vi "3d_display4.vi"() -> ()   [LabVIEW 2009]
doc: "This example demonstrates some fundamental concepts for the 3D picture control. Concepts covered include:\n\n-Object creation\n-Texturing\n-Object movement\n-Object hierarchy"
uses:
  labWOOOO/wiimotestate.ctl
  labWOOOO/wiimoteState(IR).ctl
  <vilib>/Utility/miscctls.llb/LVRectTypeDef.ctl
  <vilib>/Utility/miscctls.llb/LV3DPointTypeDef.ctl
  C:/Documents and Settings/pbooth/My Documents/labWOOOO/WiimoteLib.dll
  <vilib>/picture/3D Picture Control/NI_3D Picture Control.lvlib
  <vilib>/Analysis/NI_AALBase.lvlib
panel:
  out "Boolean":bool
  out "element x":sgl
  out "element y":sgl
  out "Cluster":cluster{"Wiimote State":T1, "IRState":T2} {"IRState"."Mode" items=["Off"=0, "Basic"=1, "Extended"=3, "Full"=5]}
  out "xadd":dbl
  out "zadd":dbl
  out "raw pitot":dbl
  in  "Calibrate pitot":bool
  in  "voltage offset":dbl=2.5
  in  "velocity scale":dbl=100.0
  in  "Set Start Time (s)":dbl
  in  "X":dbl
  in  "Z":dbl
  in  "Calibrate Z":bool
  in  "Calibrate Y":bool
  in  "Calibrate X":bool
  out "angle 2":dbl
  out "angle 1":dbl
  out "X mean acceleration":dbl format="%0.4f"
  out "Y mean acceleration":dbl format="%0.4f"
  out "X mean volts":dbl format="%0.4f"
  out "Y mean volts":dbl format="%0.4f"
  out "Z mean acceleration":dbl format="%0.4f"
  out "Z mean volts":dbl format="%0.4f"
  in  "z gain":dbl=5.0
  in  "z offset":dbl=1.25
  in  "y gain":dbl=5.0
  in  "y offset":dbl=1.25
  in  "x gain":dbl=5.0
  in  "x offset":dbl=1.25
  in  "Render Dest":enum16{"Scene Window", "Scene Display"}(ring)
  in  "Camera Controller":enum16{"None", "Spherical", "Flying"}(ring)=enum."Spherical"
  out "Scene Display":refnum<vi>(3d-picture)
  in  "stop":bool
  # "Accelerometers"
  # "Buttons"
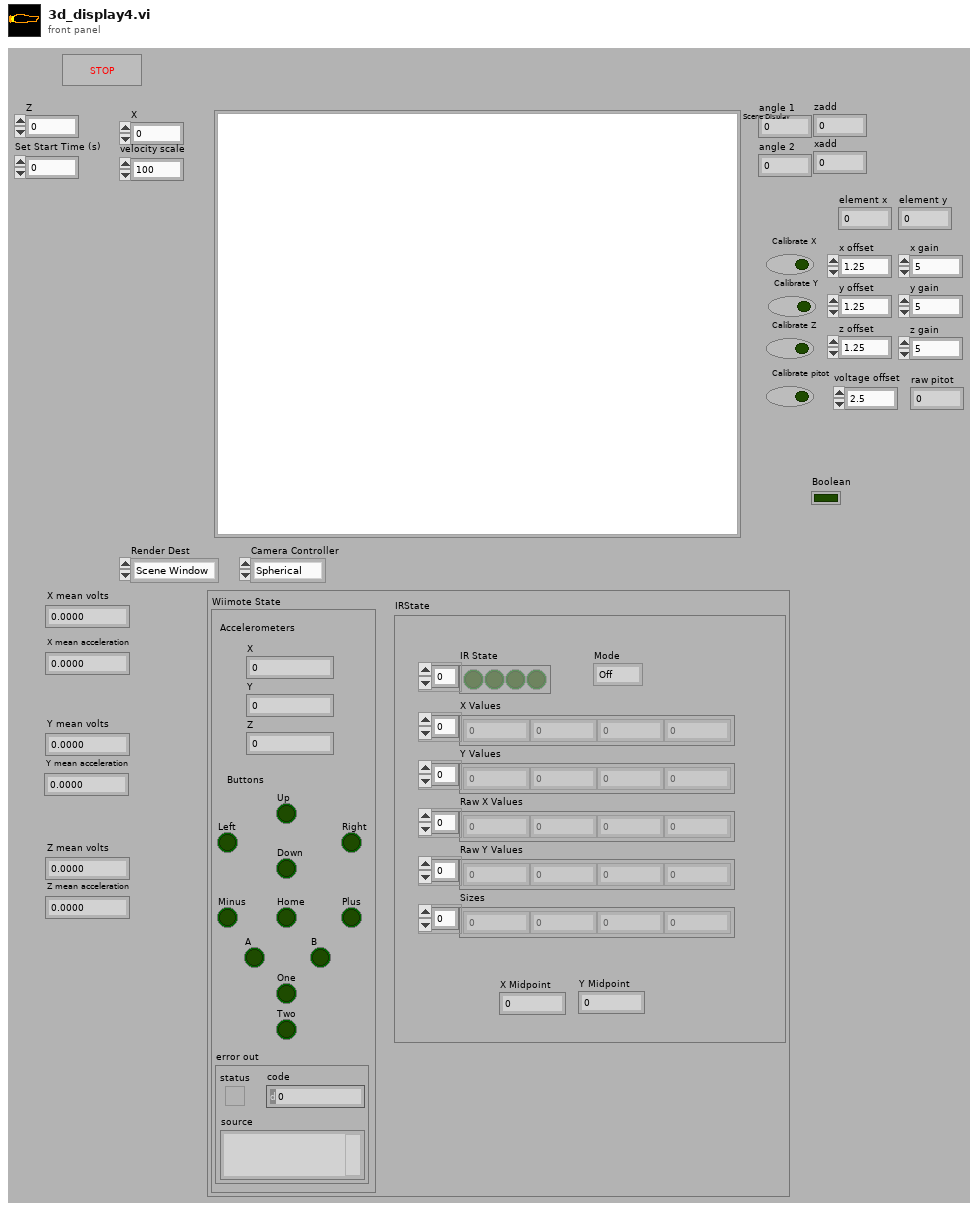
[diagram p1: front panel]
types:
  T1 = typedef "wiimotestate.ctl" = cluster{"X":sgl, "Y":sgl, "Z":sgl, "A":bool, "B":bool, "Down":bool, "Home":bool, "Left":bool, "Minus":bool, "One":bool, "Plus":bool, "Right":bool, "Two":bool, "Up":bool, "error out":errorcluster}
  T2 = typedef "wiimoteState(IR).ctl" = cluster{"Mode":u8, "IR State":bool[], "X Values":sgl[], "Y Values":sgl[], "Raw X Values":i32[], "Raw Y Values":i32[], "Sizes":i32[], "X Midpoint":sgl, "Y Midpoint":sgl}
  T3 = enum16{"As a Decal", "With Modulation", "With Blending", "As a replacement"}
  T4 = typedef "LVRectTypeDef.ctl" = cluster{"Left":i16, "Top":i16, "Right":i16, "Bottom":i16}
  T5 = enum16{"Open", "Minimized", "Maximized", "Hidden"}
  T6 = typedef "imagedata.ctl" = cluster{"image type":i32, "image depth":i32, "image":u8[], "mask":u8[], "colors":u32[], "Rectangle":cluster{"left":i16, "top":i16, "right":i16, "bottom":i16}}
  T7 = typedef "LV3DPointTypeDef.ctl" = cluster{"X":sgl, "Y":sgl, "Z":sgl}
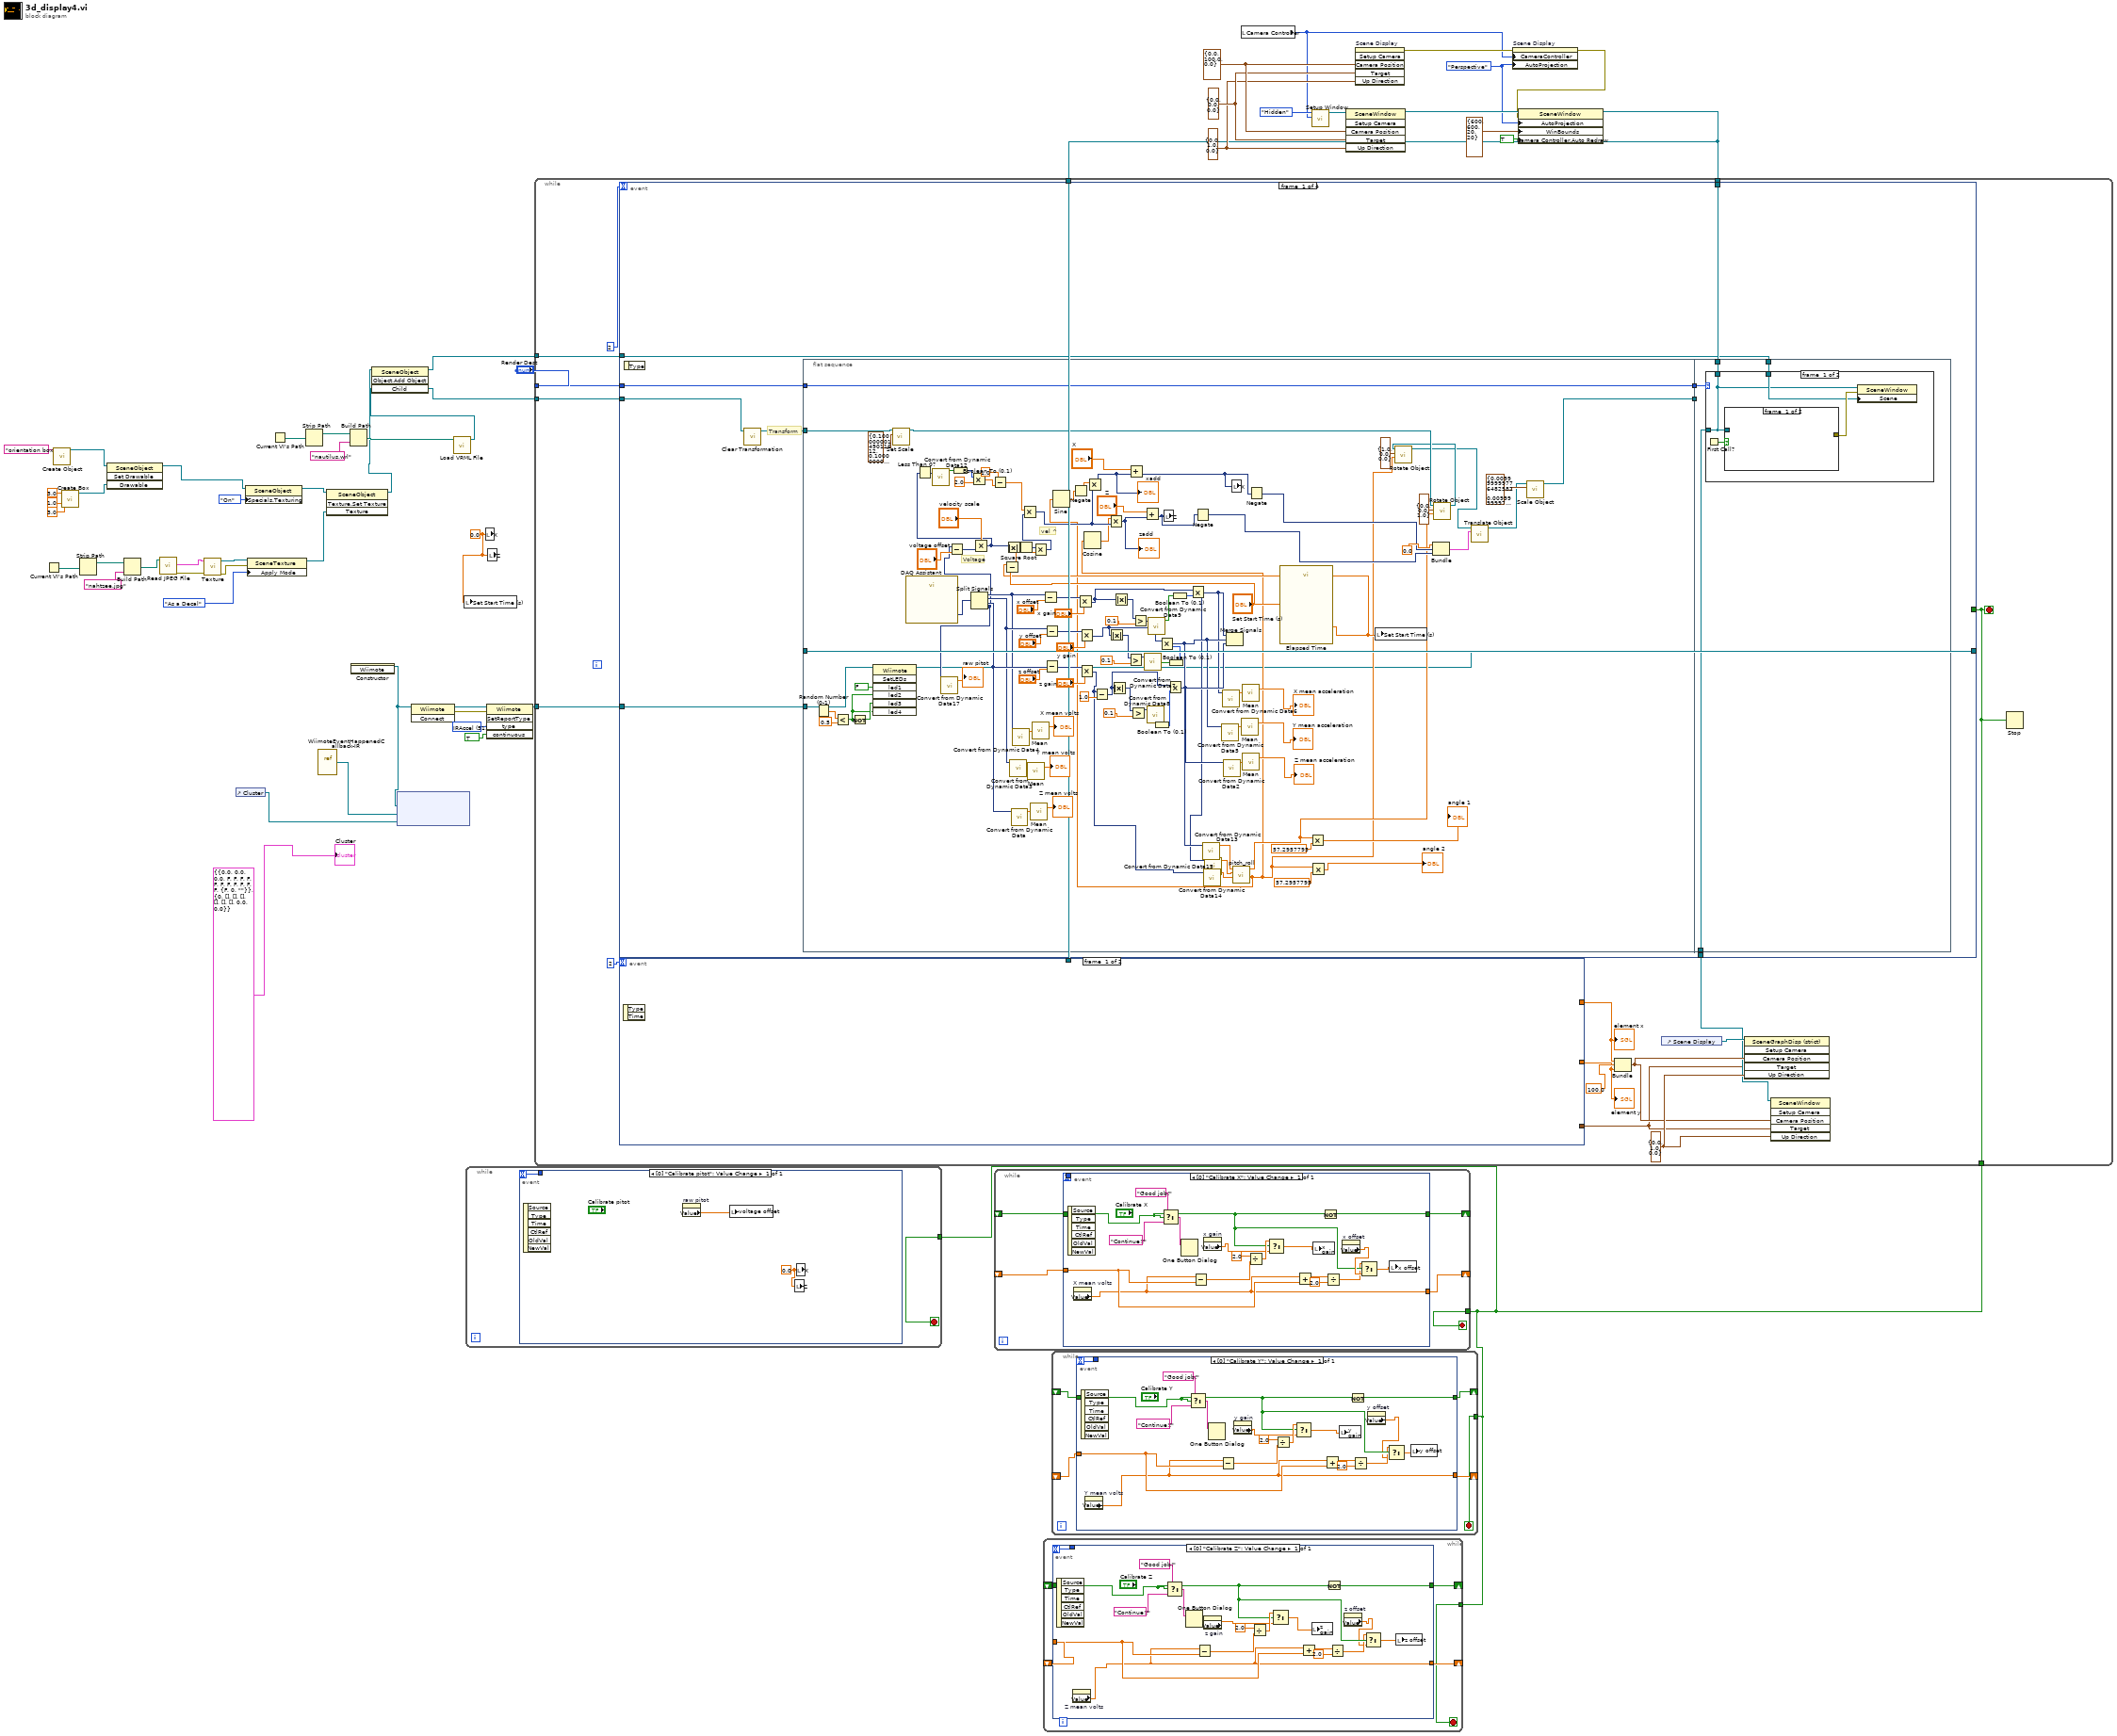
[diagram p0: block diagram]
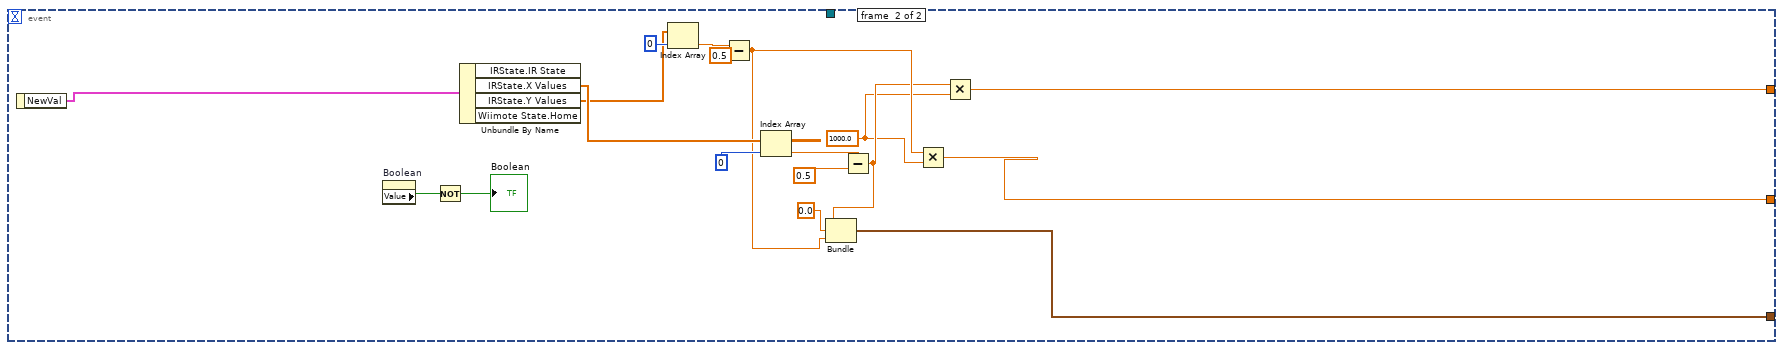
[diagram p2: hidden frame]
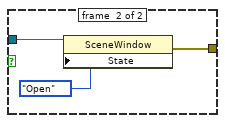
[diagram p3: hidden frame]
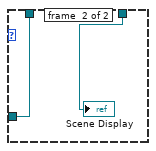
[diagram p4: hidden frame]
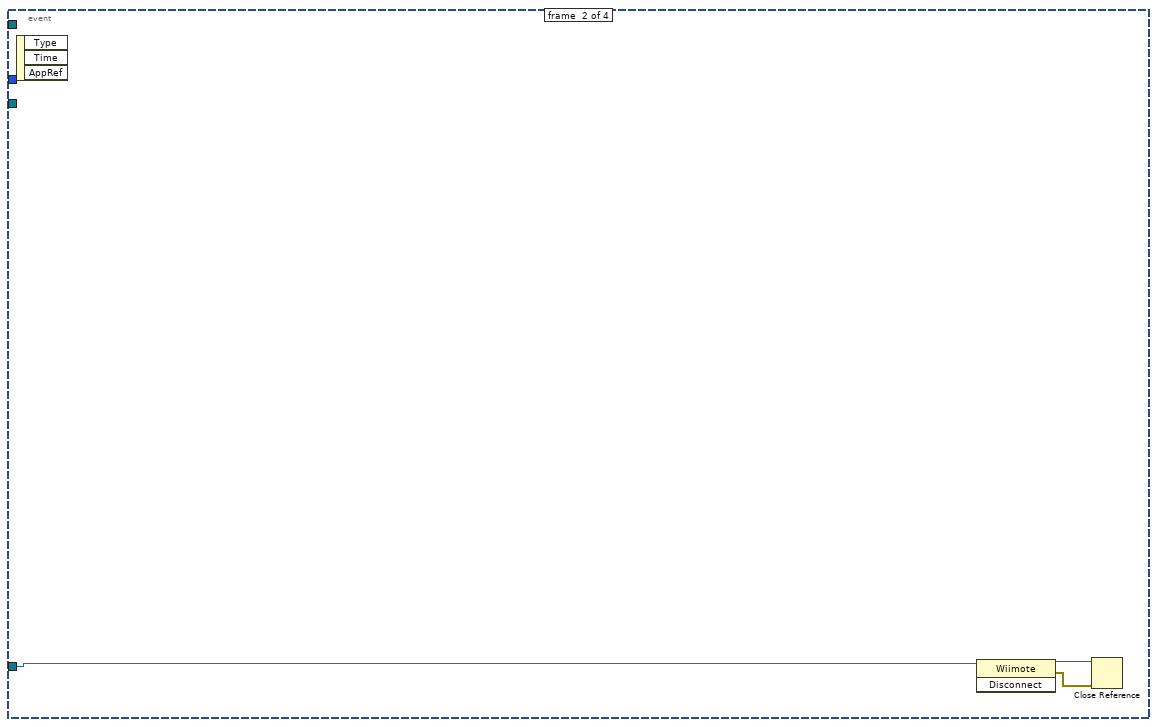
[diagram p5: hidden frame]
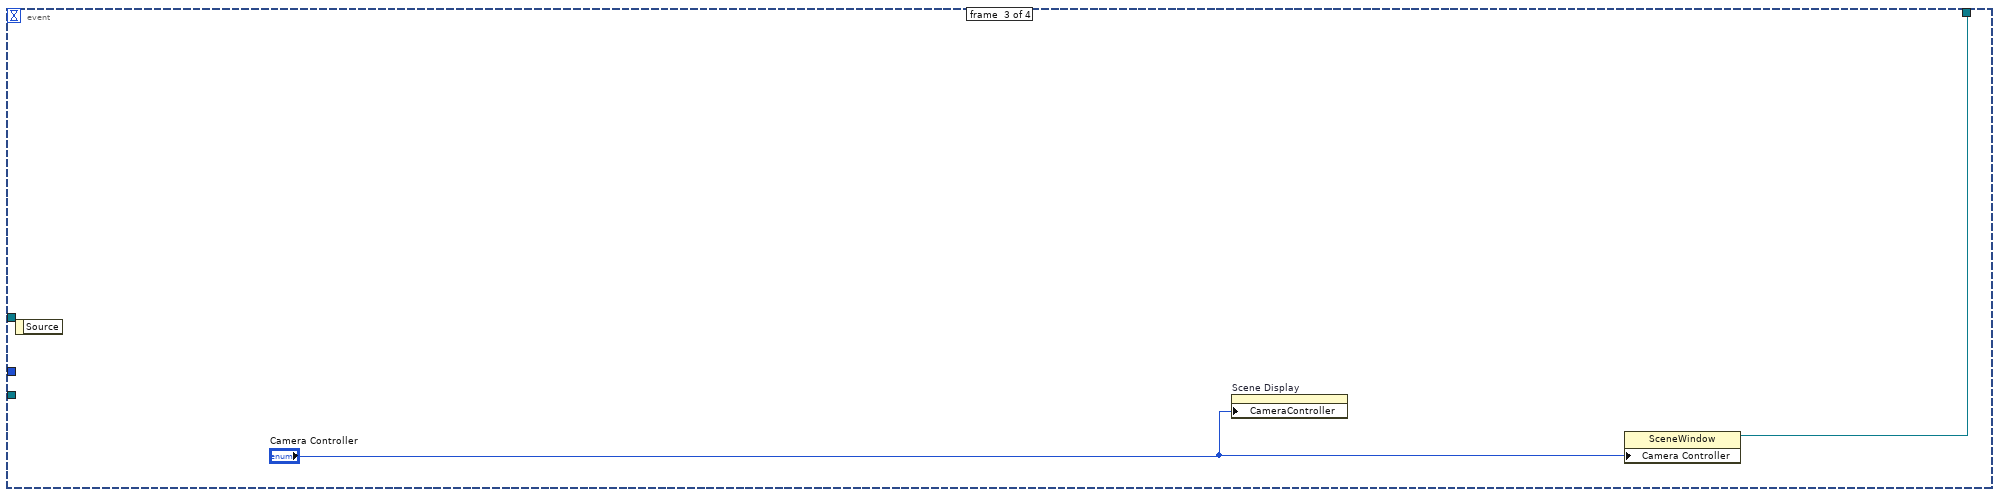
[diagram p6: hidden frame]
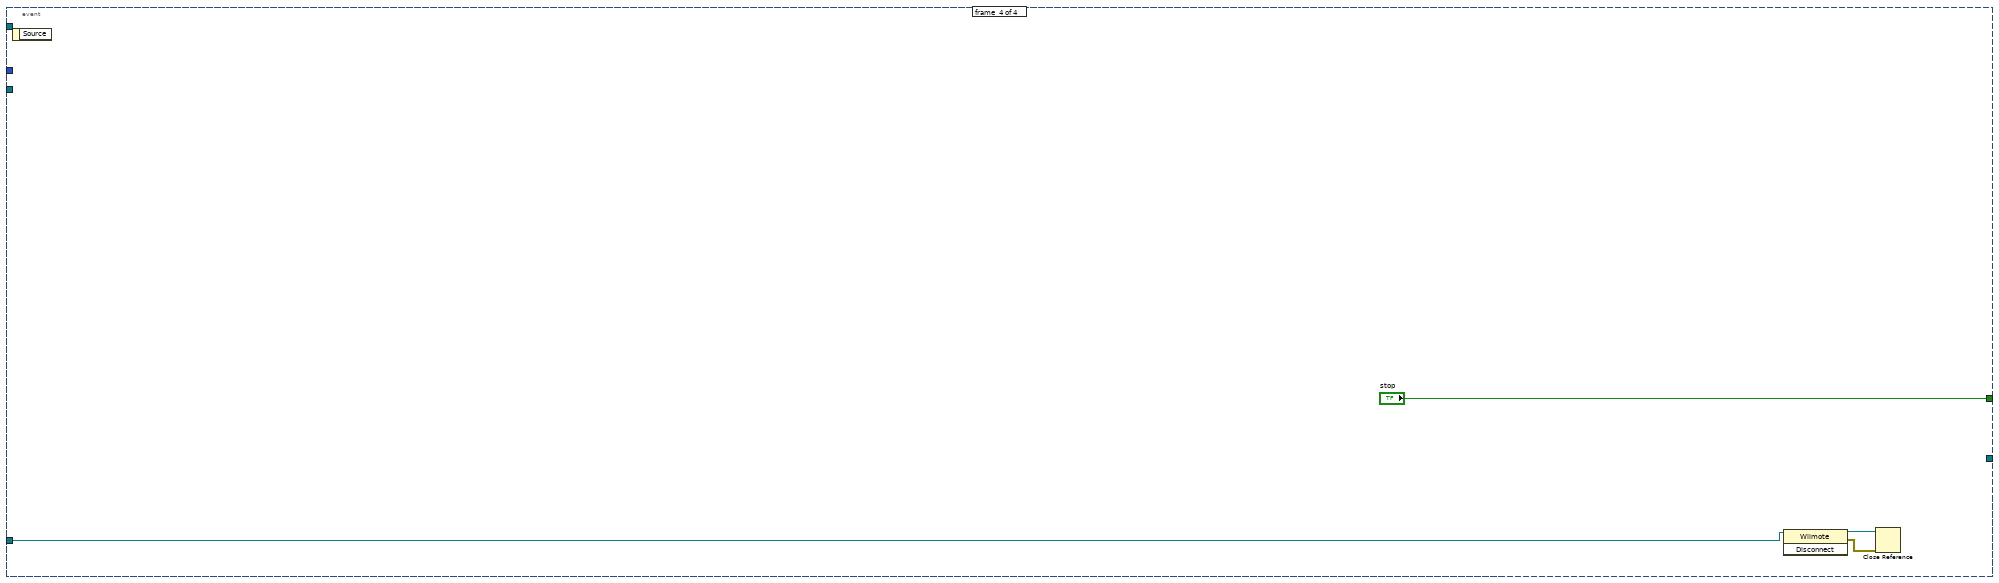
[diagram p7: hidden frame]
diagram:
  w28 = u8 51 items=["Status"=32, "ReadData"=33, "Buttons"=48, "ButtonsAccel"=49, "IRAccel"=51, "ButtonsExtension"=52, "ExtensionAccel"=53, "IRExtensionAccel"=55] ("type")
  w35 = 0.0 ("X")
  w45 = enum16{"None", "Perspective", "Orthographic"}."Perspective" ("Auto Projection Mode")
  w48 = cluster{"X":sgl, "Y":sgl, "Z":sgl} {"X"=0.0, "Y"=1.0, "Z"=0.0} ("Up Direction")
  w49 = cluster{"X":sgl, "Y":sgl, "Z":sgl} {"X"=0.0, "Y"=0.0, "Z"=0.0} ("Target")
  w50 = cluster{"X":sgl, "Y":sgl, "Z":sgl} {"X"=0.0, "Y"=100.0, "Z"=0.0} ("Camera Position")
  n1 = Current VI's Path() -> (path=w13:path)
  n2 = call <vilib>:"Create Object.vi"("Name"="orientation box") -> ("Scene:New Object"=w20:refnum<vi>)  [unwired: 9 in, 1 out]
  n3 = call <vilib>:"Create Box.vi"("Length Z"=sgl 3.0, "Length Y"=sgl 1.0, "Length X"=sgl 3.0) -> ("New Box Refnum"=w18:refnum<vi>)  [unwired: 7 in, 1 out]
  n4 = Strip Path(path=w13) -> (stripped path=w14:path)  [unwired: 1 out]
  n5 = invoke class="SceneObject" method="Set Drawable"(reference=w20, "Drawable"=w18) -> (reference out=w6:refnum<vi>)  [unwired: 2 in, 3 out]
  n6 = Build Path(base path=w14, name or relative path="nahtzee.jpg") -> (appended path=w11:path)
  n7 = call <vilib>:"Read JPEG File.vi"("path to JPEG file"=w11) -> ("error out"=w3:errorcluster, "image data"=w4:T6)  [unwired: 8 in, 1 out]
  n8 = call <vilib>:"Texture.vi"("error in (no error)"=w3, "Image"=w4) -> ("error out"=w2:errorcluster, "New Texture Refnum"=w1:refnum<vi>)  [unwired: 8 in]
  n9 = control-ref of="Cluster"() -> (w31:refnum<vi>)
  n10 = property class="SceneObject"(reference=w6, "Specials.Texturing"=enum16{"Inherit Value", "Off", "On"}."On" ("Specials:Texturing")) -> (reference out=w7:refnum<vi>)  [unwired: 1 in, 1 out]
  n11 = property class="SceneTexture"(reference=w1, error in=w2, "Apply Mode"=T3."As a Decal") -> (reference out=w9:refnum<vi>)  [unwired: 1 out]
  n12 = Current VI's Path() -> (path=w38:path)
  n13 = Strip Path(path=w38) -> (stripped path=w39:path)  [unwired: 1 out]
  n14 = vi-ref "WiimoteEventHappenedCallback-IR.vi"() -> ("vi reference"=w34:refnum<vi>)
  n15 = invoke class="SceneObject" method="Texture.Set Texture"(reference=w7, "Texture"=w9) -> (reference out=w5:refnum<vi>)  [unwired: 2 in, 3 out]
  n16 = Build Path(base path=w39, name or relative path="nautilus.wrl") -> (appended path=w36:path)
  n17 = constructor class="Wiimote"() -> (reference out=w33:refnum<k24>)  [unwired: 3 in, 2 out]
  n18 = node(w33, w34, w31) -> ()  [unwired: 2 in, 2 out]
  n19 = invoke class="Wiimote" method="Connect"(reference=w33) -> (reference out=w30:refnum<k24>, error out=w29:errorcluster)  [unwired: 2 in, 1 out]
  n20 = call <vilib>:"Load VRML File.vi"("Path"=w36) -> ("Scene:Read Scene File"=w17:refnum<vi>)  [unwired: 9 in, 1 out]
  n21 = invoke class="SceneObject" method="Object.Add Object"(reference=w5, "Child"=w17) -> (reference out=w15:refnum<vi>, "Child"=w16:refnum<vi>)  [unwired: 2 in, 2 out]
  n22 = local write "Set Start Time (s)"(w35) -> ()
  n23 = local write "X"(w35) -> ()
  n24 = invoke class="Wiimote" method="SetReportType"(reference=w30, error in=w29, "type"=w28, "continuous"=TRUE) -> (reference out=w26:refnum<k24>)  [unwired: 1 in, 4 out]
  n25 = local write "Z"(w35) -> ()
  n26 = local read "Camera Controller"() -> (w42:enum16{"None", "Spherical", "Flying"})
  n27 = call <vilib>:"Setup Window.vi"("Camera Controller"=w42, "Window State"=T5."Hidden") -> ("New Window Refnum"=w44:refnum<vi>)  [unwired: 1 in, 8 out]
  n28 = invoke class="SceneWindow" method="Setup Camera"(reference=w44, "Camera Position"=w50, "Target"=w49, "Up Direction"=w48) -> (reference out=w52:refnum<vi>)  [unwired: 2 in, 5 out]
  n29 = invoke on="Scene Display" class="SceneGraphDisp (strict)" method="Setup Camera"("Camera Position"=w50, "Target"=w49, "Up Direction"=w48) -> (error out=w47:errorcluster)  [unwired: 3 in, 5 out]
  n30 = property on="Scene Display" class="SceneGraphDisp (strict)"(error in=w47, "CameraController"=w42, "AutoProjection"=w45) -> (error out=w46:errorcluster)  [unwired: 1 in, 1 out]
  n31 = property class="SceneWindow"(reference=w52, error in=w46, "AutoProjection"=w45, "WinBounds"=T4 {"Left"=600, "Top"=600, "Right"=20, "Bottom"=20} ("Window Bounds"), "Camera Controller.Auto Redraw"=TRUE ("Camera Controller:Auto Redraw")) -> (reference out=w24:refnum<vi>)  [unwired: 1 out]
  n32 = while {
    tunnel: w24 -> [w69]
    tunnel: w16 -> [w68]
    tunnel: "Render Dest" -> [w67]
    tunnel: w26 -> [w66]
    tunnel: [w61] -> w25
    tunnel: w24 -> [w64]
    tunnel: w15 -> [w62]
    stop <- w61 stop-if-true
    w60 = T7 {"X"=0.0, "Y"=1.0, "Z"=0.0} ("Up Direction")
    n33 = event shown="[1] \"Cluster\": Value Change" {
      selector: _ -> [_ _]
      dyn-events: _ -> [_ _]
      timeout: 2 -> [_ _]
      tunnel: w64 -> [_ _]
      tunnel: [_ w72] -> w56
      tunnel: [_ w71] -> w55
      tunnel: [_ w70] -> w53
      event #0 {
        n34 = event-data() -> ()  [unwired: 1 in, 2 out]
      }
      event #1 {
        w73 = sgl 1000.0 ("y")
        n35 = event-data() -> ("NewVal"=w83:cluster{"Wiimote State":T1, "IRState":T2})  [unwired: 1 in]
        n36 = property on="Boolean" class="Bool (strict)"() -> ("Value"=w82:bool)  [unwired: 2 in, 2 out]
        n37 = Not(x=w82) -> (.not. x?=→"Boolean":bool)
        n38 = Unbundle By Name(w83) -> ("IRState.X Values"=w87:sgl[], "IRState.Y Values"=w84:sgl[])  [unwired: 2 out]
        n39 = Index Array(array=w84, index=0) -> (element=w78:sgl)
        n40 = Subtract(x=w78, y=sgl 0.5) -> (x-y=w75:sgl)
        n41 = Index Array(array=w87, index=0) -> (element=w76:sgl)
        n42 = Subtract(x=w76, y=sgl 0.5) -> (x-y=w74:sgl)
        n43 = Bundle(w74, "Y"=sgl 0.0, w75) -> (w72:cluster{sgl, "Y":sgl, sgl})  [unwired: 1 in]
        n44 = Multiply(x=w75, y=w73) -> (x*y=w70:sgl)
        n45 = Multiply(x=w74, y=w73) -> (x*y=w71:sgl)
      }
    }
    "element y" <- w53
    "element x" <- w55
    n46 = event shown="[1] Application Instance Close" {
      selector: _ -> [_ _ _ _]
      dyn-events: _ -> [_ _ _ _]
      timeout: 2 -> [_ _ _ _]
      tunnel: w69 -> [w97 _ w223 _]
      tunnel: w68 -> [w93 _ _ _]
      tunnel: [_ _ _ "stop"] -> w61
      tunnel: w67 -> [w94 _ _ _]
      tunnel: w66 -> [w91 w219 _ w225]
      tunnel: [w90 _ _ _] -> _
      tunnel: w62 -> [w89 _ _ _]
      tunnel: [w88 _ _ _] -> w57
      event #0 {
        # "Transform"
        n47 = event-data() -> ()  [unwired: 2 out]
        n48 = call <vilib>:"Clear Transformation.vi"("Object Refnum In"=w93) -> ("Object Refnum Out"=w96:refnum<vi>)  [unwired: 1 in, 9 out]
        n49 = flat-sequence {
          tunnel: w96 -> [w133]
          tunnel: [w205] -> w95
          tunnel: w94 -> [w205]
          tunnel: [w202] -> w92
          tunnel: w91 -> [w104]
          tunnel: [w98] -> w90
          tunnel: w97 -> [w209]
          tunnel: w95 -> [w208]
          tunnel: w92 -> [_]
          tunnel: w89 -> [w207]
          tunnel: [w206] -> w88
          frame #0 {
            # "vel ^"
            # "Voltage"
            n50 = Random Number (0-1)() -> (number: 0 to 1=w102:dbl)
            n51 = Less?(x=w102, y=0.5) -> (x < y?=w99:bool)
            n52 = Not(x=w99) -> (.not. x?=w100:bool)
            n53 = invoke class="Wiimote" method="SetLEDs"(reference=w104, "led1"=FALSE, "led2"=w99, "led3"=w100, "led4"=w99) -> (reference out=w98:refnum<k24>)  [unwired: 2 in, 6 out]
            n54 = call <vilib>:"Set Scale.vi"("Scale"=cluster{"X":sgl, "Y":sgl, "Z":sgl} {"X"=0.1, "Y"=0.1, "Z"=0.1}, "Scene Object"=w133) -> ("Scaled Object"=w121:refnum<vi>)  [unwired: 8 in, 1 out]
            n55 = call "DAQ Assistant"() -> ("data"=w154:dynamicdata)  [unwired: 17 in, 2 out]
            n56 = Split Signals(w154) -> (w185:dynamicdata, w187:dynamicdata, w190:dynamicdata, w117:dynamicdata)  [unwired: 4 in]
            n57 = call "Convert from Dynamic Data17"("Dynamic Data Type"=w117) -> ("Scalar"=→"raw pitot":dbl)  [unwired: 3 in]
            n58 = Subtract(x=w117, y="voltage offset") -> (x-y=w152:dynamicdata)
            n59 = Multiply(x="velocity scale", y=w152) -> (x*y=w111:dynamicdata)
            n60 = Less Than 0?(x=w111) -> (x < 0?=w110:dynamicdata)
            n61 = call "Convert from Dynamic Data12"("Dynamic Data Type"=w110) -> ("Scalar"=w143:bool)  [unwired: 3 in]
            n62 = Boolean To (0,1)(Boolean=w143) -> (0, 1=w141:i16)
            n63 = Multiply(x=w141, y=2.0) -> (x*y=w139:dbl)
            n64 = Subtract(x=1.0 ("y"), y=w139) -> (x-y=w136:dbl)
            n65 = Absolute Value(x=w111) -> (abs(x)=w138:dynamicdata)
            n66 = call "Convert from Dynamic Data3"("Dynamic Data Type"=w187) -> ("Array"=w186:dbl[])  [unwired: 3 in]
            n67 = call "Convert from Dynamic Data"("Dynamic Data Type"=w190) -> ("Array"=w192:dbl[])  [unwired: 3 in]
            n68 = call "Convert from Dynamic Data4"("Dynamic Data Type"=w185) -> ("Array"=w184:dbl[])  [unwired: 3 in]
            n69 = Square Root(x=w138) -> (sqrt(x)=w137:dynamicdata)
            n70 = call <vilib>:"Mean.vi"("X"=w186) -> ("mean"=→"Y mean volts":dbl)  [unwired: 1 out]
            n71 = call <vilib>:"Mean.vi"("X"=w192) -> ("mean"=→"Z mean volts":dbl)  [unwired: 1 out]
            n72 = call <vilib>:"Mean.vi"("X"=w184) -> ("mean"=→"X mean volts":dbl)  [unwired: 1 out]
            n73 = Subtract(x=w185, y="x offset") -> (x-y=w201:dynamicdata)
            n74 = Subtract(x=w187, y="y offset") -> (x-y=w197:dynamicdata)
            n75 = Subtract(x=w190, y="z offset") -> (x-y=w179:dynamicdata)
            n76 = Multiply(x=w201, y="x gain") -> (x*y=w160:dynamicdata)
            n77 = Multiply(x=w197, y="y gain") -> (x*y=w178:dynamicdata)
            n78 = Multiply(x=w179, y="z gain") -> (x*y=w122:dynamicdata)
            n79 = Subtract(x=w122, y=1.0) -> (x-y=w166:dynamicdata)
            n80 = Absolute Value(x=w178) -> (abs(x)=w177:dynamicdata)
            n81 = Absolute Value(x=w166) -> (abs(x)=w172:dynamicdata)
            n82 = Absolute Value(x=w160) -> (abs(x)=w165:dynamicdata)
            n83 = Greater?(x=w177, y=0.1) -> (0:w174:dynamicdata)
            n84 = Greater?(x=w172, y=0.1) -> (0:w170:dynamicdata)
            n85 = Greater?(x=w165, y=0.1) -> (0:w162:dynamicdata)
            n86 = call "Convert from Dynamic Data7"("Dynamic Data Type"=w174) -> ("Scalar"=w173:bool)  [unwired: 3 in]
            n87 = call "Convert from Dynamic Data8"("Dynamic Data Type"=w170) -> ("Scalar"=w169:bool)  [unwired: 3 in]
            n88 = call "Convert from Dynamic Data9"("Dynamic Data Type"=w162) -> ("Scalar"=w161:bool)  [unwired: 3 in]
            n89 = Boolean To (0,1)(Boolean=w169) -> (0, 1=w168:i16)
            n90 = Boolean To (0,1)(Boolean=w173) -> (0, 1=w175:i16)
            n91 = Multiply(x=w178, y=w175) -> (x*y=w124:dynamicdata)
            n92 = Multiply(x=w166, y=w168) -> (x*y=w149:dynamicdata)
            n93 = Boolean To (0,1)(Boolean=w161) -> (0, 1=w163:i16)
            n94 = Multiply(x=w160, y=w163) -> (x*y=w123:dynamicdata)
            n95 = call "Convert from Dynamic Data13"("Dynamic Data Type"=w124) -> ("Scalar"=w107:dbl)  [unwired: 3 in]
            n96 = call "Convert from Dynamic Data14"("Dynamic Data Type"=w122) -> ("Scalar"=w106:dbl)  [unwired: 3 in]
            n97 = call "Convert from Dynamic Data15"("Dynamic Data Type"=w123) -> ("Scalar"=w105:dbl)  [unwired: 3 in]
            n98 = call "Convert from Dynamic Data5"("Dynamic Data Type"=w124) -> ("Array"=w181:dbl[])  [unwired: 3 in]
            n99 = call "Convert from Dynamic Data6"("Dynamic Data Type"=w123) -> ("Array"=w180:dbl[])  [unwired: 3 in]
            n100 = call "Convert from Dynamic Data2"("Dynamic Data Type"=w149) -> ("Array"=w191:dbl[])  [unwired: 3 in]
            n101 = Merge Signals(w123, w124, w149) -> ()  [unwired: 1 out]
            n102 = call "pitch_roll.vi"("Az"=w106, "Ay"=w105, "Ax"=w107) -> ("Pitch"=w108:dbl, "Roll"=w109:dbl)  [unwired: 7 in]
            n103 = Sine(x=w108) -> (sin(x)=w112:dbl)
            n104 = Negate(x=w112) -> (-x=w113:dbl)
            n105 = Cosine(x=w108) -> (cos(x)=w131:dbl)
            n106 = call <vilib>:"Mean.vi"("X"=w181) -> ("mean"=→"Y mean acceleration":dbl)  [unwired: 1 out]
            n107 = call <vilib>:"Mean.vi"("X"=w180) -> ("mean"=→"X mean acceleration":dbl)  [unwired: 1 out]
            n108 = call <vilib>:"Mean.vi"("X"=w191) -> ("mean"=→"Z mean acceleration":dbl)  [unwired: 1 out]
            n109 = call "Elapsed Time"("Set Start Time (s)"="Set Start Time (s)") -> ("Elapsed Time (s)"=w115:dbl)  [unwired: 11 in, 7 out]
            n110 = Subtract(x=w115, y="Set Start Time (s)") -> (x-y=w144:dbl)
            n111 = Multiply(x=w137, y=w144) -> (x*y=w135:dynamicdata)
            n112 = Multiply(x=w136, y=w135) -> (x*y=w134:dynamicdata)
            n113 = Multiply(x=w113, y=w134) -> (x*y=w114:dynamicdata)
            "xadd" <- w114
            n114 = Multiply(x=w131, y=w134) -> (x*y=w148:dynamicdata)
            "zadd" <- w148
            n115 = Add(x="X", y=w114) -> (x+y=w126:dynamicdata)
            n116 = Add(x="Z", y=w148) -> (x+y=w128:dynamicdata)
            n117 = local write "Z"(w128) -> ()
            n118 = Negate(x=w128) -> (-x=w127:dynamicdata)
            n119 = local write "X"(w126) -> ()
            n120 = Negate(x=w126) -> (-x=w125:dynamicdata)
            n121 = Multiply(x=w109, y=57.2957795) -> (x*y=→"angle 1":dbl)
            n122 = Multiply(x=w108, y=57.2957795) -> (x*y=→"angle 2":dbl)
            n123 = local write "Set Start Time (s)"(w115) -> ()
            n124 = Bundle("element"=0.0, w125, w127) -> (w146:cluster{"element":dbl, dynamicdata, dynamicdata})  [unwired: 1 in]
            n125 = call <vilib>:"Rotate Object.vi"("Angle"=w109, "Axis"=cluster{"X":sgl, "Y":sgl, "Z":sgl} {"X"=0.0, "Y"=0.0, "Z"=1.0}, "Scene.Object In"=w121) -> ("Scene.Object Out"=w120:refnum<vi>)  [unwired: 7 in, 1 out]
            n126 = call <vilib>:"Rotate Object.vi"("Angle"=w108, "Axis"=cluster{"X":sgl, "Y":sgl, "Z":sgl} {"X"=1.0, "Y"=0.0, "Z"=0.0}, "Scene.Object In"=w120) -> ("Scene.Object Out"=w119:refnum<vi>)  [unwired: 7 in, 1 out]
            n127 = call <vilib>:"Translate Object.vi"("Translation"=w146, "Scene.Object In"=w119) -> ("Scene.Object Out"=w147:refnum<vi>)  [unwired: 8 in, 1 out]
            n128 = call <vilib>:"Scale Object.vi"("Scale"=cluster{"X":sgl, "Y":sgl, "Z":sgl} {"X"=0.01, "Y"=0.01, "Z"=0.01}, "Scene.Object In"=w147) -> ("Scene.Object Out"=w202:refnum<vi>)  [unwired: 8 in, 1 out]
          }
          frame #1 {
            n129 = case shown="\"Scene Window\", Default" w208 {
              tunnel: w209 -> [w210 w217]
              tunnel: w207 -> [w211 w218]
              tunnel: [w210 w217] -> w206
              frame #0 {
                n130 = First Call?() -> (First Call?: T/F=w212:bool)
                n131 = case shown="True" w212 {
                  tunnel: w210 -> [_ w216]
                  tunnel: [_ w215] -> w213
                  frame #0 {
                  }
                  frame #1 {
                    n132 = property class="SceneWindow"(reference=w216, "State"=T5."Open" ("Window State")) -> (error out=w215:errorcluster)  [unwired: 1 in, 1 out]
                  }
                }
                n133 = property class="SceneWindow"(reference=w210, error in=w213, "Scene"=w211) -> ()  [unwired: 2 out]
              }
              frame #1 {
                "Scene Display" <- w218
              }
            }
          }
        }
      }
      event #1 {
        n134 = event-data() -> ()  [unwired: 4 out]
        n135 = invoke class="Wiimote" method="Disconnect"(reference=w219) -> (reference out=w221:refnum<k24>, error out=w220:errorcluster)  [unwired: 2 in, 1 out]
        n136 = Close Reference(reference=w221, error in (no error)=w220) -> ()  [unwired: 1 out]
      }
      event #2 {
        n137 = event-data() -> ()  [unwired: 2 out]
        n138 = property on="Scene Display" class="SceneGraphDisp (strict)"("CameraController"="Camera Controller") -> ()  [unwired: 2 in, 2 out]
        n139 = property class="SceneWindow"(reference=w223, "Camera Controller"="Camera Controller") -> ()  [unwired: 1 in, 2 out]
      }
      event #3 {
        n140 = event-data() -> ()  [unwired: 2 out]
        n141 = invoke class="Wiimote" method="Disconnect"(reference=w225) -> (reference out=w227:refnum<k24>, error out=w226:errorcluster)  [unwired: 2 in, 1 out]
        n142 = Close Reference(reference=w227, error in (no error)=w226) -> ()  [unwired: 1 out]
      }
    }
    n143 = Bundle(w55, "Z"=sgl 100.0, w53) -> (w58:cluster{sgl, "Z":sgl, sgl})  [unwired: 1 in]
    n144 = control-ref of="Scene Display"() -> (w59:refnum<vi>)
    n145 = invoke on="Invoke Node" class="SceneGraphDisp (strict)" method="Setup Camera"(reference=w59, "Camera Position"=w58, "Target"=w56, "Up Direction"=w60) -> ()  [unwired: 2 in, 6 out]
    n146 = invoke class="SceneWindow" method="Setup Camera"(reference=w57, "Camera Position"=w58, "Target"=w56, "Up Direction"=w60) -> ()  [unwired: 2 in, 6 out]
    n147 = Stop(stop? (T)=w61) -> ()
  }
  n148 = while {
    tunnel: w25 -> [w228]
    stop <- w228 stop-if-true
    n149 = event shown="[0] \"Calibrate pitot\": Value Change" {
      selector: _ -> [_]
      dyn-events: _ -> [_]
      timeout: _ -> [w231]
      tunnel: [w231] -> _
      event [0] "Calibrate pitot": Value Change {
        w229 = 0.0 ("X")
        n150 = event-data() -> ()  [unwired: 1 in, 6 out]
        n151 = property on="raw pitot" class="DigNum (strict)"() -> ("Value"=w230:dbl)  [unwired: 2 in, 2 out]
        n152 = local write "voltage offset"(w230) -> ()
        n153 = local write "Z"(w229) -> ()
        n154 = local write "X"(w229) -> ()
      }
    }
  }
  n155 = while {
    shift-right: [w235] -> _
    shift-left: _ -> [w236]
    shift-right: [w234] -> _
    shift-left: _ -> [w233]
    tunnel: w25 -> [w232]
    stop <- w232 stop-if-true
    n156 = event shown="[0] \"Calibrate X\": Value Change" {
      selector: _ -> [_]
      dyn-events: _ -> [_]
      timeout: _ -> [w254]
      tunnel: [w254] -> _
      tunnel: w236 -> [w242]
      tunnel: [w250] -> w235
      tunnel: [w237] -> w234
      tunnel: w233 -> [w241]
      event [0] "Calibrate X": Value Change {
        n157 = event-data() -> ()  [unwired: 1 in, 6 out]
        n158 = property on="X mean volts" class="DigNum (strict)"() -> ("Value"=w237:dbl)  [unwired: 2 in, 2 out]
        n159 = Select(t="Good job!" ("message"), s=w242, f="Continue!!" ("message")) -> (s? t:f=w253:string)
        n160 = One Button Dialog(message=w253) -> ()  [unwired: 1 in, 1 out]
        n161 = Subtract(x=w237, y=w241) -> (x-y=w248:dbl)
        n162 = property on="x gain" class="DigNum (strict)"() -> ("Value"=w246:dbl)  [unwired: 2 in, 2 out]
        n163 = Divide(x=2.0, y=w248) -> (x/y=w247:dbl)
        n164 = Select(t=w247, s=w242, f=w246) -> (s? t:f=w245:dbl)
        n165 = Add(x=w237, y=w241) -> (x+y=w239:dbl)
        n166 = local write "x gain"(w245) -> ()
        n167 = Not(x=w242) -> (.not. x?=w250:bool)
        n168 = Divide(x=w239, y=2.0) -> (x/y=w238:dbl)
        n169 = property on="x offset" class="DigNum (strict)"() -> ("Value"=w243:dbl)  [unwired: 2 in, 2 out]
        n170 = Select(t=w238, s=w242, f=w243) -> (s? t:f=w244:dbl)
        n171 = local write "x offset"(w244) -> ()
      }
    }
  }
  n172 = while {
    shift-right: [w257] -> _
    shift-left: _ -> [w256]
    shift-right: [w259] -> _
    shift-left: _ -> [w258]
    tunnel: w25 -> [w255]
    stop <- w255 stop-if-true
    n173 = event shown="[0] \"Calibrate Z\": Value Change" {
      selector: _ -> [_]
      dyn-events: _ -> [_]
      timeout: _ -> [w277]
      tunnel: [w277] -> _
      tunnel: w258 -> [w269]
      tunnel: [w273] -> w259
      tunnel: [w260] -> w257
      tunnel: w256 -> [w268]
      event [0] "Calibrate Z": Value Change {
        n174 = event-data() -> ()  [unwired: 1 in, 6 out]
        n175 = property on="Z mean volts" class="DigNum (strict)"() -> ("Value"=w260:dbl)  [unwired: 2 in, 2 out]
        n176 = Select(t="Good job!" ("message"), s=w269, f="Continue!!" ("message")) -> (s? t:f=w276:string)
        n177 = One Button Dialog(message=w276) -> ()  [unwired: 1 in, 1 out]
        n178 = Subtract(x=w260, y=w268) -> (x-y=w271:dbl)
        n179 = property on="z gain" class="DigNum (strict)"() -> ("Value"=w263:dbl)  [unwired: 2 in, 2 out]
        n180 = Divide(x=2.0, y=w271) -> (x/y=w270:dbl)
        n181 = Select(t=w270, s=w269, f=w263) -> (s? t:f=w261:dbl)
        n182 = Add(x=w260, y=w268) -> (x+y=w266:dbl)
        n183 = local write "z gain"(w261) -> ()
        n184 = Not(x=w269) -> (.not. x?=w273:bool)
        n185 = Divide(x=w266, y=2.0) -> (x/y=w265:dbl)
        n186 = property on="z offset" class="DigNum (strict)"() -> ("Value"=w262:dbl)  [unwired: 2 in, 2 out]
        n187 = Select(t=w265, s=w269, f=w262) -> (s? t:f=w264:dbl)
        n188 = local write "z offset"(w264) -> ()
      }
    }
  }
  n189 = while {
    shift-right: [w282] -> _
    shift-left: _ -> [w281]
    shift-right: [w279] -> _
    shift-left: _ -> [w280]
    tunnel: w25 -> [w278]
    stop <- w278 stop-if-true
    n190 = event shown="[0] \"Calibrate Y\": Value Change" {
      selector: _ -> [_]
      dyn-events: _ -> [_]
      timeout: _ -> [w300]
      tunnel: [w300] -> _
      tunnel: w281 -> [w292]
      tunnel: [w296] -> w282
      tunnel: [w283] -> w279
      tunnel: w280 -> [w291]
      event [0] "Calibrate Y": Value Change {
        n191 = event-data() -> ()  [unwired: 1 in, 6 out]
        n192 = property on="Y mean volts" class="DigNum (strict)"() -> ("Value"=w283:dbl)  [unwired: 2 in, 2 out]
        n193 = Select(t="Good job!" ("message"), s=w292, f="Continue!!" ("message")) -> (s? t:f=w299:string)
        n194 = One Button Dialog(message=w299) -> ()  [unwired: 1 in, 1 out]
        n195 = Subtract(x=w283, y=w291) -> (x-y=w294:dbl)
        n196 = property on="y gain" class="DigNum (strict)"() -> ("Value"=w287:dbl)  [unwired: 2 in, 2 out]
        n197 = Divide(x=2.0, y=w294) -> (x/y=w293:dbl)
        n198 = Select(t=w293, s=w292, f=w287) -> (s? t:f=w286:dbl)
        n199 = Add(x=w283, y=w291) -> (x+y=w289:dbl)
        n200 = local write "y gain"(w286) -> ()
        n201 = Not(x=w292) -> (.not. x?=w296:bool)
        n202 = Divide(x=w289, y=2.0) -> (x/y=w288:dbl)
        n203 = property on="y offset" class="DigNum (strict)"() -> ("Value"=w285:dbl)  [unwired: 2 in, 2 out]
        n204 = Select(t=w288, s=w292, f=w285) -> (s? t:f=w284:dbl)
        n205 = local write "y offset"(w284) -> ()
      }
    }
  }
  "Cluster" <- cluster{"Wiimote State":T1, "IRState":T2} {"Wiimote State"={"X"=0.0, "Y"=0.0, "Z"=0.0, "A"=FALSE, "B"=FALSE, "Down"=FALSE, "Home"=FALSE, "Left"=FALSE, "Minus"=FALSE, "One"=FALSE, "Plus"=FALSE, "Right"=FALSE, "Two"=FALSE, "Up"=FALSE, "error out"={"status"=FALSE, "code"=0, "source"=""}}, "IRState"={"Mode"=0, "IR State"=[], "X Values"=[], "Y Values"=[], "Raw X Values"=[], "Raw Y Values"=[], "Sizes"=[], "X Midpoint"=0.0, "Y Midpoint"=0.0}} ("Cluster")
